vi "ADC Read Volts.vi"(8 "error in (no error)":errorcluster, 10 "ADC Channel Selection":T1, 11 "LINX-ADS1X15 in":refnum<class "LINX-ADS1256.lvclass">) -> (0 "error out":errorcluster, 2 "ADC Volts":dbl, 3 "LINX-ADS1X15 out":refnum<class "LINX-ADS1256.lvclass">)   [LabVIEW 2020, in "LINX-ADS1256.lvclass"]
uses:
  LINX-ADS1256.lvclass
  Channel Selection.ctl
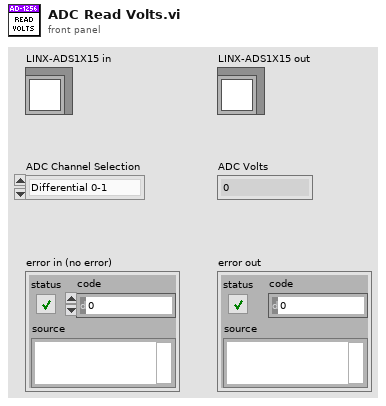
[diagram p1: front panel]
types:
  T1 = typedef "LINX-ADS1256.lvclass/Channel Selection.ctl" = enum16{"Differential 0-1", "Differential 2-3", "Single Ended 0", "Single Ended 1", "Single Ended 2", "Single Ended 3"}
  T2 = typedef "LINX-ADS1256.lvclass/Programmable Gain Selection.ctl" = enum16{"+/-5V (1)", "+/-2.5V (2)", "+/-1.25V (4)", "+/-0.625V (8)", "+/-312.5mV (16)", "+/-156.25mV (32)", "+/-78.125mV (64)"}
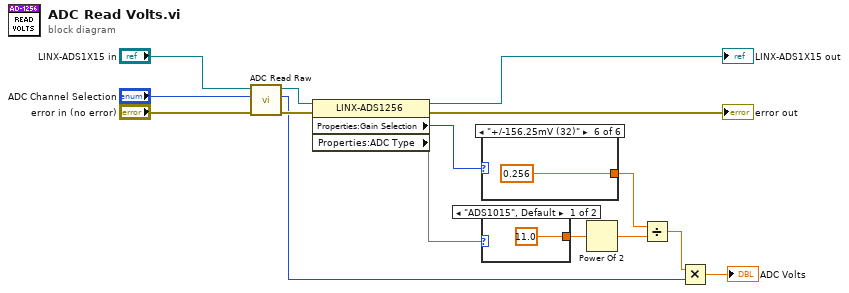
[diagram p0: block diagram]
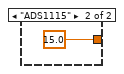
[diagram p2: hidden frame]
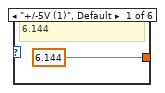
[diagram p3: hidden frame]
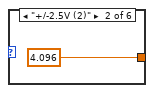
[diagram p4: hidden frame]
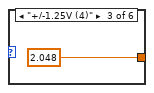
[diagram p5: hidden frame]
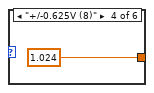
[diagram p6: hidden frame]
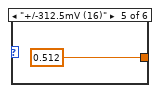
[diagram p7: hidden frame]
diagram:
  n1 = call-dynamic "ADC Read Raw.vi"("error in (no error)"="error in (no error)", "ADC Channel Selection"="ADC Channel Selection", "LINX-ADS1X15 in"="LINX-ADS1X15 in") -> ("error out"=w10:errorcluster, "ADC Raw"=w3:i16, "LINX-ADS1X15 out"=w15:refnum<class "LINX-ADS1256.lvclass">)  [unwired: 6 in]
  n2 = property class="LINX-ADS1256"(reference=w15, error in=w10) -> (reference out=→"LINX-ADS1X15 out":refnum<class "LINX-ADS1256.lvclass">, error out=→"error out":errorcluster, "Properties:Gain Selection"=w8:T2, "Properties:ADC Type"=w1)
  n3 = case shown="\"+/-156.25mV (32)\"" w8 {
    tunnel: [6.144 4.096 2.048 1.024 0.512 0.256] -> w6
    frame "+/-5V (1)", Default {
      # "6.144"
    }
    frame "+/-2.5V (2)" {
    }
    frame "+/-1.25V (4)" {
    }
    frame "+/-0.625V (8)" {
    }
    frame "+/-312.5mV (16)" {
    }
    frame "+/-156.25mV (32)" {
    }
  }
  n4 = case shown="\"ADS1015\", Default" w1 {
    tunnel: [11.0 ("x") 15.0 ("x")] -> w7
    frame "ADS1015", Default {
    }
    frame "ADS1115" {
    }
  }
  n5 = Power Of 2(x=w7) -> (2^x=w5:dbl)
  n6 = Divide(x=w6, y=w5) -> (x/y=w4:dbl)
  n7 = Multiply(x=w4, y=w3) -> (x*y=→"ADC Volts":dbl)
